vi "클릭반응시간.vi"() -> ()   [LabVIEW 2014]
panel:
  out "시간측정":dbl
  in  "정지":bool
  in  "확인 버튼":bool
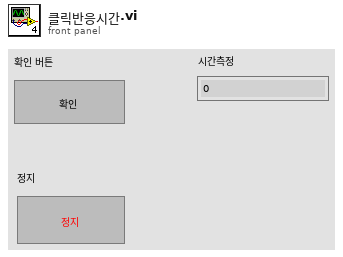
[diagram p1: front panel]
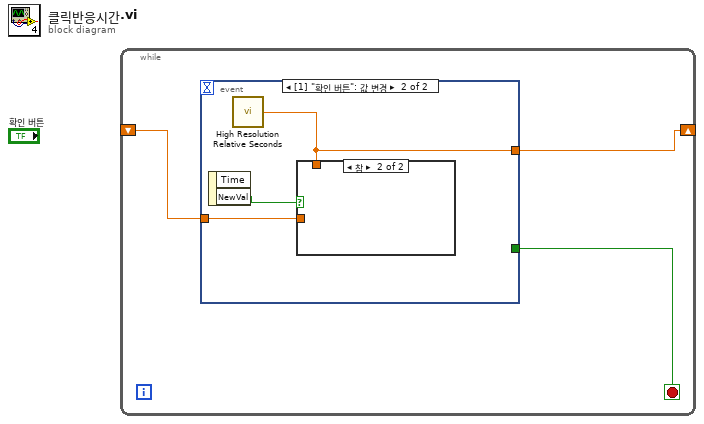
[diagram p0: block diagram]
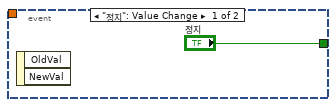
[diagram p2: hidden frame]
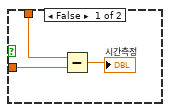
[diagram p3: hidden frame]
diagram:
  n1 = while {
    shift-right: [w2] -> _
    shift-left: _ -> [w1]
    stop <- w3 stop-if-true
    n2 = event shown="[1] \"확인 버튼\": 값 변경" {
      selector: _ -> [_ _]
      dyn-events: _ -> [_ _]
      timeout: _ -> [_ _]
      tunnel: ["정지" _] -> w3
      tunnel: [_ w5] -> w2
      tunnel: w1 -> [_ w6]
      event "정지": Value Change {
        n3 = event-data() -> ()  [unwired: 1 in, 2 out]
      }
      event "확인 버튼": Value Change {
        n4 = event-data() -> ("NewVal"=w7:bool)  [unwired: 1 in, 1 out]
        n5 = call <vilib>:"High Resolution Relative Seconds.vi"() -> ("relative seconds"=w5:dbl)
        n6 = case shown="참" w7 {
          tunnel: w5 -> [w10 _]
          tunnel: w6 -> [w9 _]
          frame False {
            n7 = Subtract(x=w10, y=w9) -> (x-y=→"시간측정":dbl)
          }
          frame True {
          }
        }
      }
    }
  }
